vi "HB_CloseLog.vi"(8 "error in (no error)":errorcluster, 11 "HBDeviceRef":T1) -> (0 "error out":errorcluster, 3 "HBDeviceRef":T1)   [LabVIEW 2016]
doc: "Closes the currently opened file on the Huskie Board. If no file is opened, invoking this VI has no effect."
uses:
  <vilib>/Rock Robotics/WPI/SerialPort/WPI_SerialPortRef.ctl
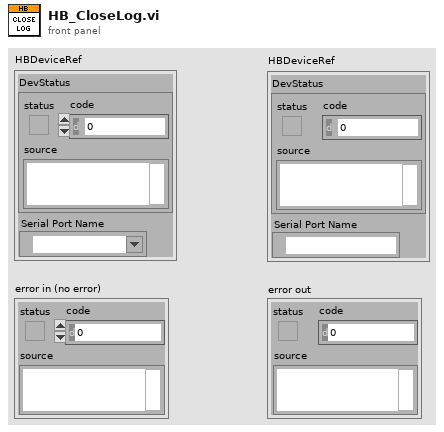
[diagram p1: front panel]
types:
  T1 = typedef "WPI_SerialPortRef.ctl" = cluster{"DevStatus":errorcluster, "Serial Port Name":refnum<visa-resource-name>}
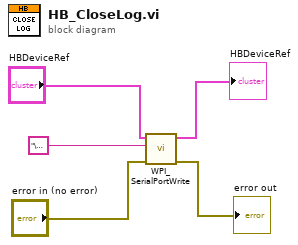
[diagram p0: block diagram]
diagram:
  n1 = call <vilib>:"WPI_SerialPortWrite.vi"("error in (no error)"="error in (no error)", "Buffer"="\u0004", "SerialPortRef"="HBDeviceRef") -> ("error out"=→"error out":errorcluster, "SerialPortRef"=→"HBDeviceRef":T1)  [unwired: 6 in, 1 out]
